vi "Html Report.vi"(0 "标题配置":cluster{"title":string, "font":T1}={"title"="智能农业小车数据监测报告", "font"={"font name"="", "font size"=24.0, "bold"=2, "italic"=2, "underline"=2, "strike through"=2, "font color"=16777222}} {"font"."font size" format="%0.2f"; "font"."strike through" items=["Unchanged", "Yes", "No"]; "font"."underline" items=["Unchanged", "Yes", "No"]; "font"."italic" items=["Unchanged", "Yes", "No"]; "font"."bold" items=["Unchanged", "Yes", "No"]}, 1 "报表信息":cluster{"font":T1, "字符串":string}={"font"={"font name"="", "font size"=12.0, "bold"=2, "italic"=2, "underline"=2, "strike through"=2, "font color"=16777222}, "字符串"=""} {"font"."font size" format="%0.2f"; "font"."strike through" items=["Strk Unchanged", "Strk Yes", "Strk No"]; "font"."underline" items=["Und Unchanged", "Und Yes", "Und No"]; "font"."italic" items=["Ital Unchanged", "Ital Yes", "Ital No"]; "font"."bold" items=["Bold Unchanged", "Bold Yes", "Bold No"]}, 2 "文本":cluster{"font":T1, "字符串":string}={"font"={"font name"="", "font size"=12.0, "bold"=2, "italic"=2, "underline"=2, "strike through"=2, "font color"=16777222}, "字符串"=""} {"font"."font size" format="%0.2f"; "font"."strike through" items=["Strk Unchanged", "Strk Yes", "Strk No"]; "font"."underline" items=["Und Unchanged", "Und Yes", "Und No"]; "font"."italic" items=["Ital Unchanged", "Ital Yes", "Ital No"]; "font"."bold" items=["Bold Unchanged", "Bold Yes", "Bold No"]}, 3 "表格":T2={"auto format"=11, "font"={"font name"="", "font size"=0.0, "bold"=0, "italic"=0, "underline"=0, "strike through"=0, "font color"=0}, "表格 2"=[]} {"auto format" items=["xlRangeAutoFormat3DEffects1"=13, "xlRangeAutoFormat3DEffects2"=14, "xlRangeAutoFormatAccounting1"=4, "xlRangeAutoFormatAccounting2"=5, "xlRangeAutoFormatAccounting3"=6, "xlRangeAutoFormatAccounting4"=17, "xlRangeAutoFormatClassic1"=1, "xlRangeAutoFormatClassic2"=2, "xlRangeAutoFormatClassic3"=3, "xlRangeAutoFormatColor1"=7, "xlRangeAutoFormatColor2"=8, "xlRangeAutoFormatColor3"=9, "xlRangeAutoFormatList1"=10, "xlRangeAutoFormatList2"=11, "xlRangeAutoFormatList3"=12, "xlRangeAutoFormatLocalFormat1"=15, "xlRangeAutoFormatLocalFormat2"=16, "xlRangeAutoFormatLocalFormat3"=19, "xlRangeAutoFormatLocalFormat4"=20, "xlRangeAutoFormatReport1"=21, "xlRangeAutoFormatReport2"=22, "xlRangeAutoFormatReport3"=23, "xlRangeAutoFormatReport4"=24, "xlRangeAutoFormatReport5"=25, "xlRangeAutoFormatReport6"=26, "xlRangeAutoFormatReport7"=27, "xlRangeAutoFormatReport8"=28, "xlRangeAutoFormatReport9"=29, "xlRangeAutoFormatReport10"=30, "xlRangeAutoFormatClassicPivotTable"=31, "xlRangeAutoFormatTable1"=32, "xlRangeAutoFormatTable2"=33, "xlRangeAutoFormatTable3"=34, "xlRangeAutoFormatTable4"=35, "xlRangeAutoFormatTable5"=36, "xlRangeAutoFormatTable6"=37, "xlRangeAutoFormatTable7"=38, "xlRangeAutoFormatTable8"=39, "xlRangeAutoFormatTable9"=40, "xlRangeAutoFormatTable10"=41, "xlRangeAutoFormatPTNone"=42, "xlRangeAutoFormatNone"=-4142, "xlRangeAutoFormatSimple"=-4154]; "font"."font size" format="%0.2f"; "font"."strike through" items=["Strk Unchanged", "Strk Yes", "Strk No"]; "font"."underline" items=["Und Unchanged", "Und Yes", "Und No"]; "font"."italic" items=["Ital Unchanged", "Ital Yes", "Ital No"]; "font"."bold" items=["Bold Unchanged", "Bold Yes", "Bold No"]}, 4 "图表配置":T4={"chart type"=4, "graph title (\"\")"="环境数据"} {"chart type" items=["xlColumnClustered"=51, "xlColumnStacked"=52, "xlColumnStacked100"=53, "xl3DColumnClustered"=54, "xl3DColumnStacked"=55, "xl3DColumnStacked100"=56, "xlBarClustered"=57, "xlBarStacked"=58, "xlBarStacked100"=59, "xl3DBarClustered"=60, "xl3DBarStacked"=61, "xl3DBarStacked100"=62, "xlLineStacked"=63, "xlLineStacked100"=64, "xlLineMarkers"=65, "xlLineMarkersStacked"=66, "xlLineMarkersStacked100"=67, "xlPieOfPie"=68, "xlPieExploded"=69, "xl3DPieExploded"=70, "xlBarOfPie"=71, "xlXYScatterSmooth"=72, "xlXYScatterSmoothNoMarkers"=73, "xlXYScatterLines"=74, "xlXYScatterLinesNoMarkers"=75, "xlAreaStacked"=76, "xlAreaStacked100"=77, "xl3DAreaStacked"=78, "xl3DAreaStacked100"=79, "xlDoughnutExploded"=80, "xlRadarMarkers"=81, "xlRadarFilled"=82, "xlSurface"=83, "xlSurfaceWireframe"=84, "xlSurfaceTopView"=85, "xlSurfaceTopViewWireframe"=86, "xlBubble"=15, "xlBubble3DEffect"=87, "xlStockHLC"=88, "xlStockOHLC"=89, "xlStockVHLC"=90, "xlStockVOHLC"=91, "xlCylinderColClustered"=92, "xlCylinderColStacked"=93, "xlCylinderColStacked100"=94, "xlCylinderBarClustered"=95, "xlCylinderBarStacked"=96, "xlCylinderBarStacked100"=97, "xlCylinderCol"=98, "xlConeColClustered"=99, "xlConeColStacked"=100, "xlConeColStacked100"=101, "xlConeBarClustered"=102, "xlConeBarStacked"=103, "xlConeBarStacked100"=104, "xlConeCol"=105, "xlPyramidColClustered"=106, "xlPyramidColStacked"=107, "xlPyramidColStacked100"=108, "xlPyramidBarClustered"=109, "xlPyramidBarStacked"=110, "xlPyramidBarStacked100"=111, "xlPyramidCol"=112, "xl3DColumn"=-4100, "xlLine"=4, "xl3DLine"=-4101, "xl3DPie"=-4102, "xlPie"=5, "xlXYScatter"=-4169, "xl3DArea"=-4098, "xlArea"=1, "xlDoughnut"=-4120, "xlRadar"=-4151]}, 5 "环境数据":dbl[](graph), 6 "报告类型":u16(ring), 7 "簇":T3={"Save Report 2"=FALSE, "路径"=path "/Report.html", "Print Report 2"=FALSE, "份数"=1} {"份数" min=1 max=10 step=1}, 8 "当前报警":i32(listbox)=-1) -> ()   [LabVIEW 2012]
uses:
  <vilib>/addons/_office/_wordsub.llb/font.ctl
  <vilib>/Utility/NIReport.llb/NI_report.lvclass
  <vilib>/Utility/NIReport.llb/Append Report Text (str wrap).vi
  <vilib>/printing/OpenHTMLReport.llb/Open HTML Report in Browser (Refnum).vi
  <vilib>/Utility/NIReport.llb/NI_ReportGenerationCore.lvlib
panel:
  out "表格 2":string[][](table)
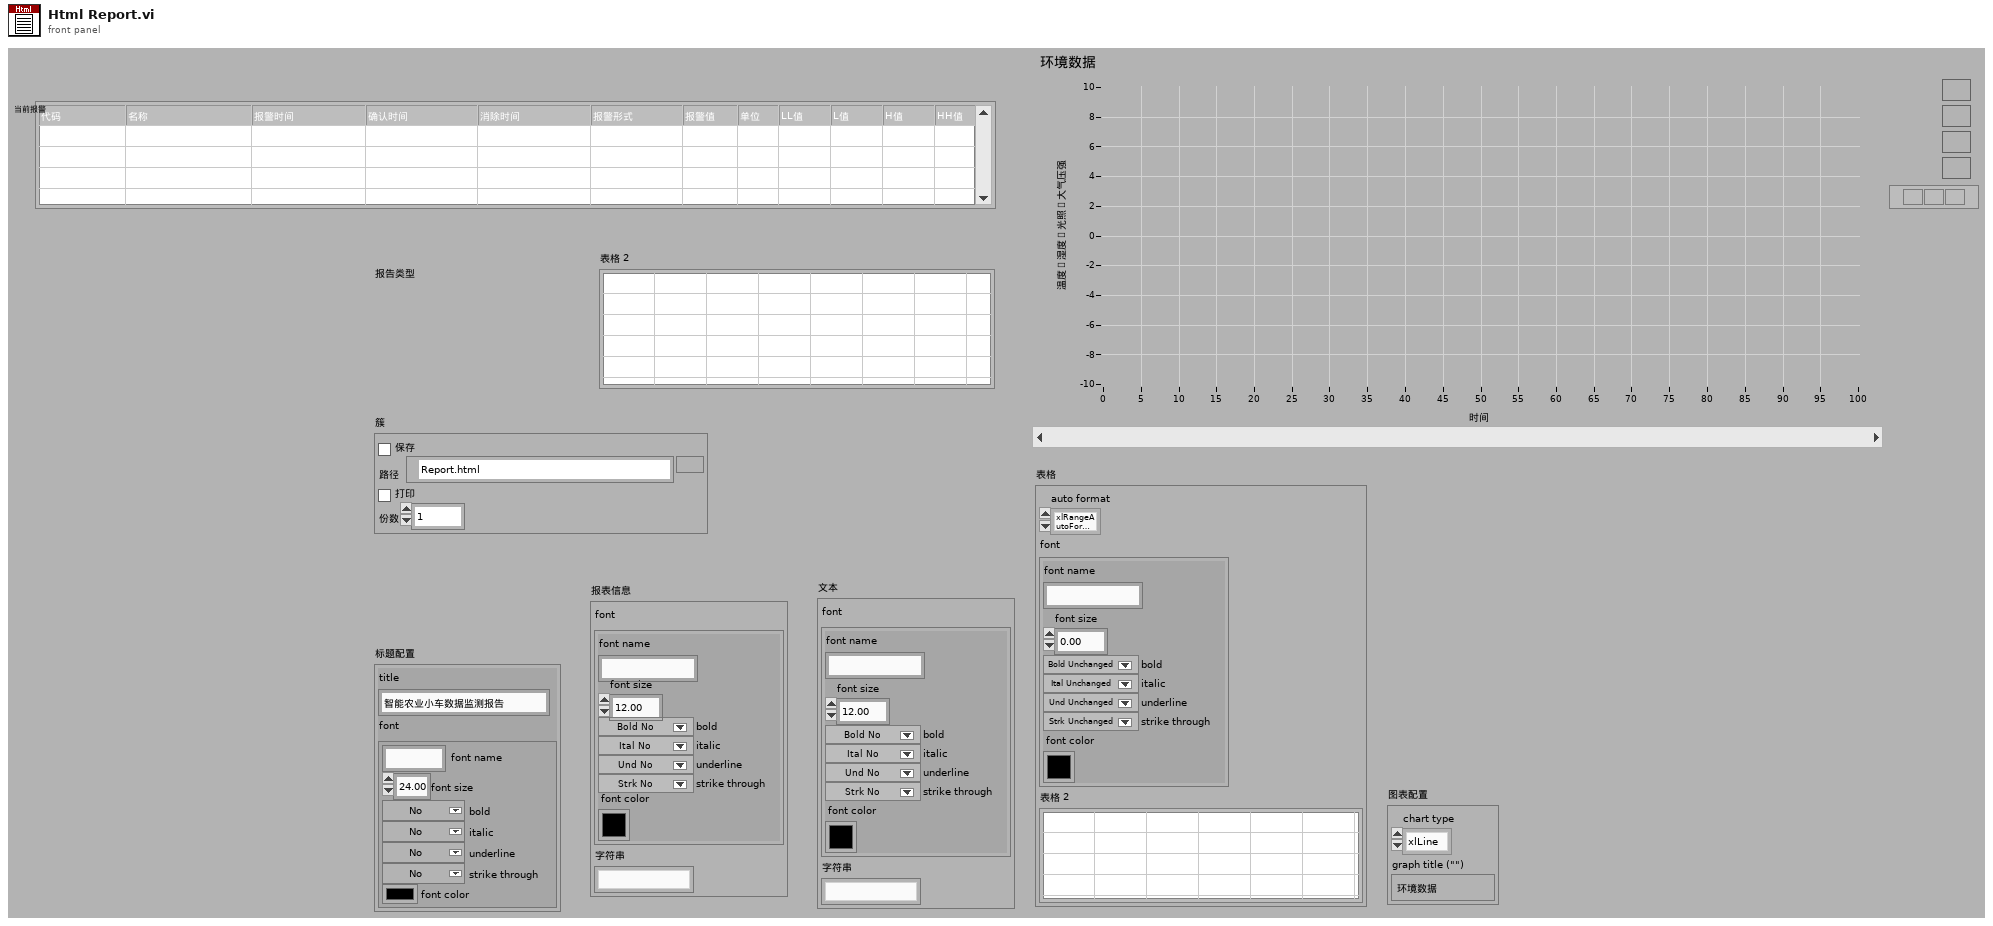
[diagram p1: front panel]
types:
  T1 = typedef "font.ctl" = cluster{"font name":string, "font size":dbl, "bold":u16, "italic":u16, "underline":u16, "strike through":u16, "font color":u32}
  T2 = cluster{"auto format":i32, "font":T1, "表格 2":string[][]}
  T3 = cluster{"Save Report 2":bool, "路径":path, "Print Report 2":bool, "份数":i32}
  T4 = cluster{"chart type":i32, "graph title (\"\")":string}
  T5 = cluster{"Charset (-1)":i16, "Weight (-1)":i16, "Name":string, "Size":string}
  T6 = cluster{"Italic":enum16{"Italic Unchanged", "Italic On", "Italic Off"}, "Strike Through":enum16{"Strike Through Unchanged", "Strike Through On", "Strike Through Off"}, "Underline":enum16{"Underline Unchanged", "Underline On", "Underline Off"}, "Bold":enum16{"Bold Unchanged", "Bold On", "Bold Off"}}
  T7 = typedef "Generate Report Object Reference.ctl" = refnum<class "NI_report.lvclass">
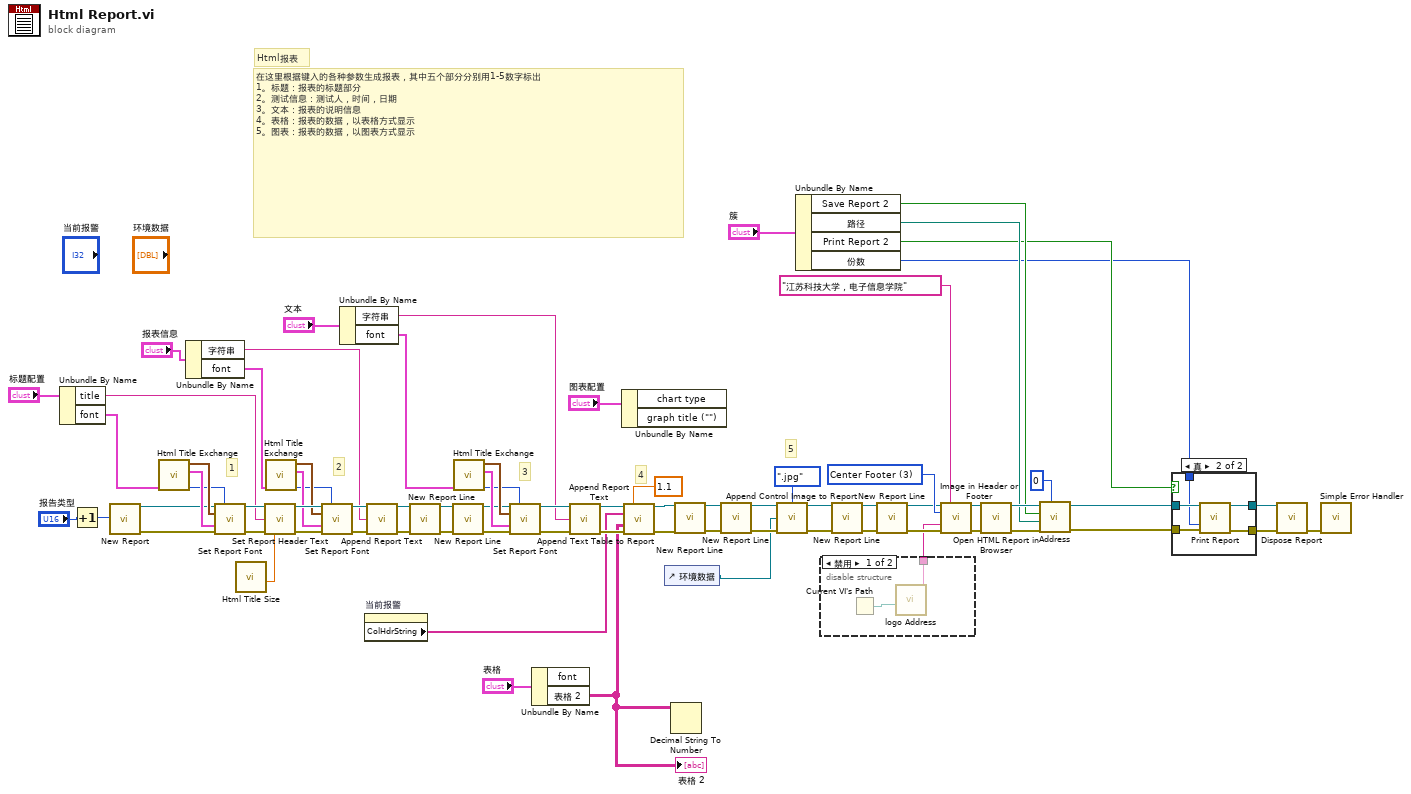
[diagram p0: block diagram]
diagram:
  w62 = u16 3 items=["Left Header", "Left Footer", "Center Header", "Center Footer", "Right Herader", "Right Footer"] ("select header or footer")
  # "3"
  # "2"
  # "5"
  # "4"
  # "1"
  # "Html报表"
  # "在这里根据键入的各种参数生成报表，其中五个部分分别用1-5数字标出\n1。标题：报表的标题部分\n2。测试信息：测试人，时间，日期\n3。文本：报表的说明信息\n4。表格：报表的数据，以表格方式显示\n5。图表：报表的数据，以图表方式显示"
  n1 = Unbundle By Name("标题配置") -> ("title"=w13:string, "font"=w14:T1)
  n2 = Increment(x="报告类型") -> (x+1=w72:u16)
  n3 = call <vilib>:"New Report.vi"("report type"=w72) -> ("report out"=w16:refnum<class "NI_report.lvclass">, "error out"=w15:errorcluster)  [unwired: 13 in]
  n4 = call "Html Title Exchange.vi"("font"=w14) -> ("text color (unchanged)"=w37:u32, "font settings"=w63:T5, "text options"=w64:T6)  [unwired: 8 in]
  n5 = Unbundle By Name("报表信息") -> ("字符串"=w11:string, "font"=w12:T1)
  n6 = call-dynamic "Set Report Font.vi"("report in"=w16, "text color (unchanged)"=w37, "text options"=w64, "font settings"=w63, "error in (no error)"=w15) -> ("report out"=w65:refnum<class "NI_report.lvclass">, "error out"=w66:errorcluster)  [unwired: 8 in, 1 out]
  n7 = call "Html Title Size.vi"() -> ("数值"=w40:dbl)  [unwired: 11 in]
  n8 = call-dynamic "Set Report Header Text.vi"("report in"=w65, "center header text"=w13, "error in (no error)"=w66, "HTML header size"=w40) -> ("report out"=w67:refnum<class "NI_report.lvclass">, "error out"=w68:errorcluster)  [unwired: 10 in]
  n9 = call "Html Title Exchange.vi"("font"=w12) -> ("text color (unchanged)"=w36:u32, "font settings"=w38:T5, "text options"=w39:T6)  [unwired: 8 in]
  n10 = call-dynamic "Set Report Font.vi"("report in"=w67, "text color (unchanged)"=w36, "text options"=w39, "font settings"=w38, "error in (no error)"=w68) -> ("report out"=w69:refnum<class "NI_report.lvclass">, "error out"=w26:errorcluster)  [unwired: 8 in, 1 out]
  n11 = Unbundle By Name("文本") -> ("字符串"=w10:string, "font"=w9:T1)
  n12 = property on="当前报警" class="MCListbox (严格)"() -> ("ColHdrString"=w2:string[])  [unwired: 2 in, 2 out]
  n13 = call-poly <vilib>:"Append Report Text.vi"("report in"=w69, "text"=w11, "error in (no error)"=w26) -> ("report out"=w47:refnum<class "NI_report.lvclass">, "error out"=w48:errorcluster)  [unwired: 9 in, 2 out]
  n14 = call-dynamic "New Report Line.vi"("report in"=w47, "error in (no error)"=w48) -> ("report out"=w30:refnum<class "NI_report.lvclass">, "error out"=w27:errorcluster)  [unwired: 12 in]
  n15 = call-dynamic "New Report Line.vi"("report in"=w30, "error in (no error)"=w27) -> ("report out"=w29:refnum<class "NI_report.lvclass">, "error out"=w28:errorcluster)  [unwired: 12 in]
  n16 = call "Html Title Exchange.vi"("font"=w9) -> ("text color (unchanged)"=w31:u32, "font settings"=w32:T5, "text options"=w33:T6)  [unwired: 8 in]
  n17 = call-dynamic "Set Report Font.vi"("report in"=w29, "text color (unchanged)"=w31, "text options"=w33, "font settings"=w32, "error in (no error)"=w28) -> ("report out"=w49:refnum<class "NI_report.lvclass">, "error out"=w50:errorcluster)  [unwired: 8 in, 1 out]
  n18 = Unbundle By Name("表格") -> ("表格 2"=w7:string[][])  [unwired: 1 out]
  "表格 2" <- w7
  n19 = call-poly <vilib>:"Append Report Text.vi"("report in"=w49, "text"=w10, "error in (no error)"=w50) -> ("report out"=w46:refnum<class "NI_report.lvclass">, "error out"=w45:errorcluster)  [unwired: 9 in, 2 out]
  n20 = Unbundle By Name("图表配置") -> ()  [unwired: 2 out]
  n21 = call-dynamic "Append Text Table to Report.vi"("report in"=w46, "column width (1)"=1.1, "column headers"=w2, "text data"=w7, "error in (no error)"=w45) -> ("report out"=w60:refnum<class "NI_report.lvclass">, "error out"=w59:errorcluster)  [unwired: 7 in, 2 out]
  n22 = control-ref of="环境数据"() -> (w1:refnum<vi>)
  n23 = Decimal String To Number(string=w7) -> ()  [unwired: 2 in, 2 out]
  n24 = call-dynamic "New Report Line.vi"("report in"=w60, "error in (no error)"=w59) -> ("report out"=w43:refnum<class "NI_report.lvclass">, "error out"=w44:errorcluster)  [unwired: 12 in]
  n25 = call-dynamic "New Report Line.vi"("report in"=w43, "error in (no error)"=w44) -> ("report out"=w51:refnum<class "NI_report.lvclass">, "error out"=w52:errorcluster)  [unwired: 12 in]
  n26 = call-dynamic "Append Control Image to Report.vi"("report in"=w51, "image file type (.jpg)"=enum16{".jpg", ".png"}.".jpg" ("image file type(.png)"), "ctrl reference"=w1, "error in (no error)"=w52) -> ("report out"=w54:refnum<class "NI_report.lvclass">, "error out"=w55:errorcluster)  [unwired: 8 in, 2 out]
  n27 = Unbundle By Name("簇") -> ("Save Report 2"=w6:bool, "路径"=w5:path, "Print Report 2"=w4:bool, "份数"=w3:i32)
  n28 = disable-structure shown="禁用" {
    disable-tunnel: [w77 _] -> w22
    frame Disabled {
      n29 = Current VI's Path() -> (path=w78:path)
      n30 = call "logo Address.vi"("path"=w78) -> ("字符串"=w77:string)  [unwired: 10 in]
    }
    frame Enabled {
    }
  }
  n31 = call-dynamic "New Report Line.vi"("report in"=w54, "error in (no error)"=w55) -> ("report out"=w58:refnum<class "NI_report.lvclass">, "error out"=w57:errorcluster)  [unwired: 12 in]
  n32 = call-dynamic "New Report Line.vi"("report in"=w58, "error in (no error)"=w57) -> ("report out"=w42:refnum<class "NI_report.lvclass">, "error out"=w41:errorcluster)  [unwired: 12 in]
  n33 = call-dynamic "Image in Header or Footer.vi"("report in"=w42, "select header or footer"=w62, "image path"=w22, "error in (no error)"=w41, "text above image"="江苏科技大学，电子信息学院" ("right footer text")) -> ("report out"=w34:refnum<class "NI_report.lvclass">, "error out"=w35:errorcluster)  [unwired: 9 in]
  n34 = call-poly <vilib>:"Open HTML Report in Browser.vi"("report in"=w34, "error in (no error)"=w35) -> ("report out"=w21:refnum<class "NI_report.lvclass">, "error out"=w20:errorcluster)  [unwired: 11 in, 1 out]
  n35 = call "Address.vi"("报告类型"=u16 0 ("报告类型 2"), "错误簇输入"=w20, "路径"=w5, "保存？"=w6, "报告输入"=w21) -> ("错误簇输出"=w19:errorcluster, "报告输出"=w18:T7)  [unwired: 5 in]
  n36 = case shown="真" w4 {
    tunnel: [w80 w84] -> w25
    tunnel: [w79 w85] -> w24
    tunnel: w19 -> [w79 w83]
    tunnel: w18 -> [w80 w82]
    tunnel: w3 -> [_ w81]
    frame False {
    }
    frame True {
      n37 = call-dynamic "Print Report.vi"("report in"=w82, "number of copies (1)"=w81, "error in (no error)"=w83) -> ("report out"=w84:T7, "error out"=w85:errorcluster)  [unwired: 11 in]
    }
  }
  n38 = call-dynamic "Dispose Report.vi"("report in"=w25, "error in (no error)"=w24) -> ("error out"=w23:errorcluster)  [unwired: 13 in]
  n39 = call <vilib>:"Simple Error Handler.vi"("error in (no error)"=w23) -> ()  [unwired: 4 in, 5 out]
